vi "CommandServoPosition.vi"(7 "Debug with FS control? (F)":bool, 8 "Error in":errorcluster, 9 "position [%FS]":dbl(slide) scale=-200.0..200.0, 11 "PWM Ref In":T3) -> (0 "Error out":errorcluster)   [LabVIEW 2013]
doc: "This VI takes in a rudder setpoint in the RudderSuggestedSetpoint typedef (range of -1 to 1) and turns it into a a servo position. It is also passed a zero reference so that the rudder can be reinitialized to a new zero.\n\nAssumptions: there is a bound on the range of the rudder inside of this VI, set in consultation with the ME team. A zero position is also passed into this VI, which then translates an incoming -1 (full port) into the zero position minus half of the bounded range.\n\nThe 'Debug with FS Control?' boolean is made for TestRudderServo.vi, so the user can twiddle the servo around without any 'degrees to servo units' conversion. This should be used with new servos to get the 'degrees to servo units' conversion right.\n\nEric Schneider, March 2014"
uses:
  <vilib>/myRIO/Instrument Drivers/Onboard IO/PWM/typedefs/PWM Reference.ctl
  <vilib>/myRIO/Common/Instrument Driver Framework/Utilities/typedefs/myRIO Generic Hardware Reference.ctl
  <vilib>/myRIO/Common/Instrument Driver Framework/Utilities/typedefs/Hardware Version Enum.ctl
  <vilib>/myRIO/Common/Instrument Driver Framework/Utilities/typedefs/myRIO v1.0 Reference.ctl
  <vilib>/myRIO/Common/Instrument Driver Framework/Utilities/typedefs/Generic FPGA Reference.ctl
  <vilib>/myRIO/Common/Instrument Driver Framework/myRIO v1.0/PWM/typedefs/PWM Channels Enum.ctl
  <vilib>/myRIO/Instrument Drivers/Onboard IO/PWM/typedefs/PWM Configuration.ctl
  Data/TypeDefs/Notifiers.ctl
  Data/TypeDefs/UTM Location.ctl
  Data/TypeDefs/Sail Set Suggestions.ctl
  Data/TypeDefs/Rudder Set Suggestions.ctl
  Data/TypeDefs/OverrideInformation.ctl
  Data/TypeDefs/OverrideMode.ctl
  Data/TypeDefs/MotorSetup.ctl
  Data/TypeDefs/DynamixelSetupInfo.ctl
  <vilib>/myRIO/Common/Instrument Driver Framework/myRIO v1.0/PWM/vis/myRIO v1.0 Write PWM.vi
  <vilib>/Utility/error.llb/Error Cluster From Error Code.vi
  <vilib>/myRIO/Instrument Drivers/Onboard IO/PWM/PWM.lvlib
panel:
  out "Rudder Command":T1 min=-1.0 max=1.0 scale=1.0..-1.0
  in  "NotifierReff":T2
  in  "%FS per degree":dbl=1.85 format="%#_13g"
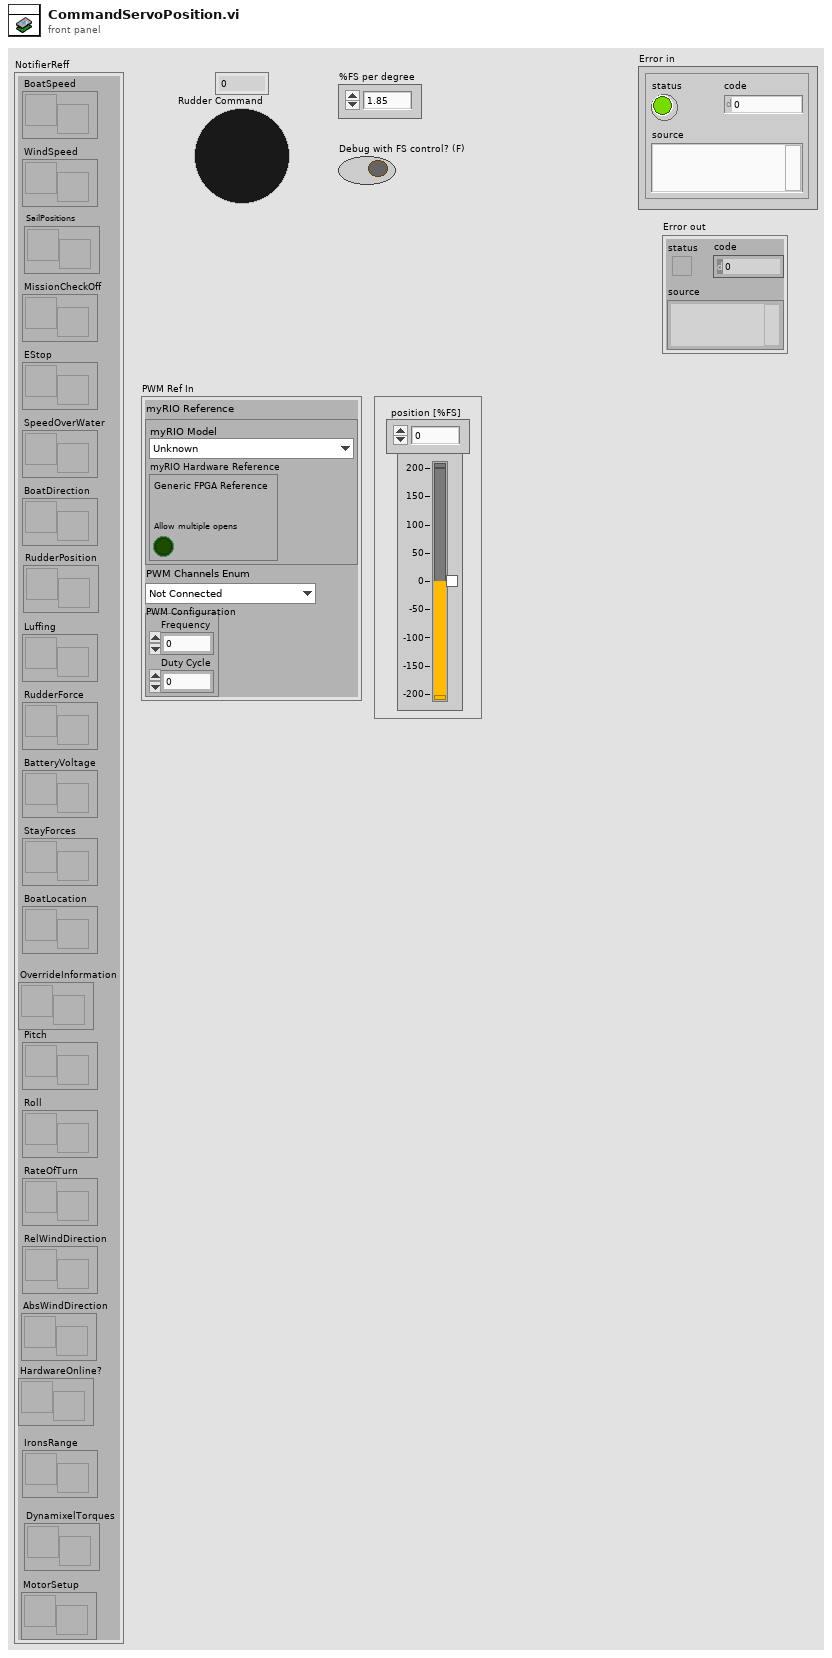
[diagram p1: front panel]
types:
  T1 = typedef "Rudder Set Suggestions.ctl" = dbl
  T2 = typedef "Notifiers.ctl" = cluster{"BoatSpeed":refnum<notifier>, "WindSpeed":refnum<notifier>, "MissionCheckOff":refnum<notifier>, "EStop":refnum<notifier>, "SpeedOverWater":refnum<notifier>, "BoatDirection":refnum<notifier>, "Luffing":refnum<notifier>, "RudderForce":refnum<notifier>, "BatteryVoltage":refnum<notifier>, "StayForces":refnum<notifier>, "BoatLocation":refnum<notifier>, "Pitch":refnum<notifier>, "Roll":refnum<notifier>, "RateOfTurn":refnum<notifier>, "RelWindDirection":refnum<notifier>, "SailPositions":refnum<notifier>, "RudderPosition":refnum<notifier>, "IronsRange":refnum<notifier>, "AbsWindDirection":refnum<notifier>, "OverrideInformation":refnum<notifier>, "DynamixelTorques":refnum<notifier>, "HardwareOnline?":refnum<notifier>, "MotorSetup":refnum<notifier>}
  T3 = typedef "PWM.lvlib/PWM Reference.ctl" = cluster{"myRIO Reference":T4, "PWM Channels Enum":T8, "PWM Configuration":T9}
  T4 = typedef "myRIO Generic Hardware Reference.ctl" = cluster{"myRIO Model":T5, "myRIO Hardware Reference":T6}
  T5 = typedef "Hardware Version Enum.ctl" = enum16{"Unknown", "myRIO-1900", "myRIO-1950"}
  T6 = typedef "myRIO v1.0 Reference.ctl" = cluster{"Generic FPGA Reference":T7, "Allow multiple opens":bool}
  T7 = typedef "Generic FPGA Reference.ctl" = refnum<k20>
  T8 = typedef "PWM Channels Enum.ctl" = enum16{"Not Connected", "C/PWM0", "C/PWM1", "A/PWM0", "A/PWM1", "A/PWM2", "B/PWM0", "B/PWM1", "B/PWM2"}
  T9 = typedef "PWM.lvlib/PWM Configuration.ctl" = cluster{"Frequency":dbl, "Duty Cycle":dbl}
  T10 = typedef "MotorSetup.ctl" = cluster{"Rudder Trim (FS Units)":dbl, "Rudder Range (deg)":dbl, "Main Dynamixel Set Data":T11, "Jib Dynamixel Set Data":T11}
  T11 = typedef "DynamixelSetupInfo.ctl" = cluster{"Lower Winch Bound":dbl, "Upper Winch Bound":dbl, "Reverse Winch Direction?":bool, "Dynamixel Cycle Number":i32}
  T12 = typedef "OverrideInformation.ctl" = cluster{"OverrideMode":T13, "SailSetting":T14, "Suggested Rudder Setpoint":T1}
  T13 = typedef "OverrideMode.ctl" = enum16{"None", "Rudder", "Sails", "Both"}
  T14 = typedef "Sail Set Suggestions.ctl" = cluster{"MainSailSuggestion":dbl, "JibSailSuggestion":dbl}
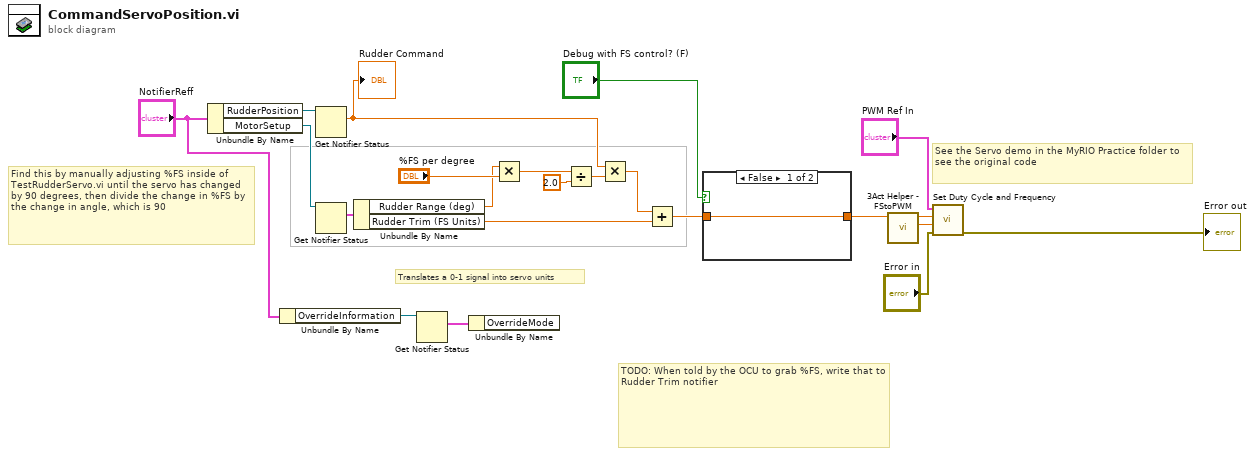
[diagram p0: block diagram]
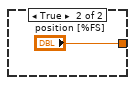
[diagram p2: hidden frame]
diagram:
  # "TODO: When told by the OCU to grab %FS, write that to Rudder Trim notifier"
  # "Translates a 0-1 signal into servo units"
  # "Find this by manually adjusting %FS inside of TestRudderServo.vi until the servo has changed by 90 degrees, then divide the change in %FS by the change in angle, which is 90"
  # "See the Servo demo in the MyRIO Practice folder to see the original code"
  n1 = Unbundle By Name("NotifierReff") -> ("RudderPosition"=w11:refnum<notifier>, "MotorSetup"=w12:refnum<notifier>)
  n2 = Unbundle By Name("NotifierReff") -> ("OverrideInformation"=w2:refnum<notifier>)
  n3 = Get Notifier Status(notifier=w11) -> (current notification=w9:T1)  [unwired: 1 in, 4 out]
  "Rudder Command" <- w9
  n4 = Get Notifier Status(notifier=w12) -> (current notification=w10:T10)  [unwired: 1 in, 4 out]
  n5 = Unbundle By Name(w10) -> ("Rudder Range (deg)"=w5:dbl, "Rudder Trim (FS Units)"=w4:dbl)
  n6 = Get Notifier Status(notifier=w2) -> (current notification=w1:T12)  [unwired: 1 in, 4 out]
  n7 = Unbundle By Name(w1) -> ()  [unwired: 1 out]
  n8 = Multiply(x=w5, y="%FS per degree") -> (x*y=w17:dbl)
  n9 = Divide(x=w17, y=2.0) -> (x/y=w16:dbl)
  n10 = Multiply(x=w9, y=w16) -> (x*y=w15:T1)
  n11 = Add(x=w15, y=w4) -> (x+y=w14:T1)
  n12 = case shown="False" "Debug with FS control? (F)" {
    tunnel: [w23 "position [%FS]"] -> w8
    tunnel: w14 -> [w23 _]
    frame False {
    }
    frame True {
    }
  }
  n13 = call "3Act Helper - FStoPWM.vi"("Suggested Rudder Setpoint in"=w8) -> ("freq [Hz] out"=w6:dbl, "Suggested Rudder Setpoint out"=w7:T1)  [unwired: 9 in]
  n14 = call <vilib>:"Set Duty Cycle and Frequency.vi"("error in (no error)"="Error in", "Frequency (Hz)"=w6, "Duty Cycle (0-1)"=w7, "PWM Ref In"="PWM Ref In") -> ("error out"=→"Error out":errorcluster)  [unwired: 5 in, 1 out]
